vi "Comm visa sync.vi"(8 "error in (no error)":errorcluster, 10 "Command":u8[](array[numeric]), 11 "VISA in":refnum<visa-resource-name>="COM7") -> (0 "error out":errorcluster, 1 "sync info":string, 2 "Response":string, 3 "VISA out":refnum<visa-resource-name>)   [LabVIEW 2014, in "AISAS motor.lvclass"]
uses:
  AISAS motor.lvclass
  <vilib>/Instr/_visa.llb/VISA Flush IO Buffer Mask.ctl
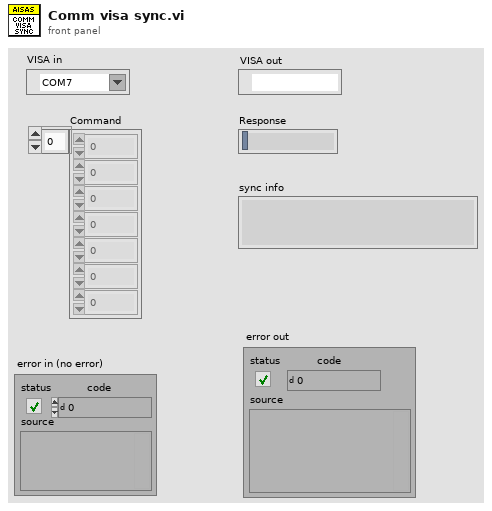
[diagram p1: front panel]
types:
  T1 = typedef "VISA Flush IO Buffer Mask.ctl" = u16
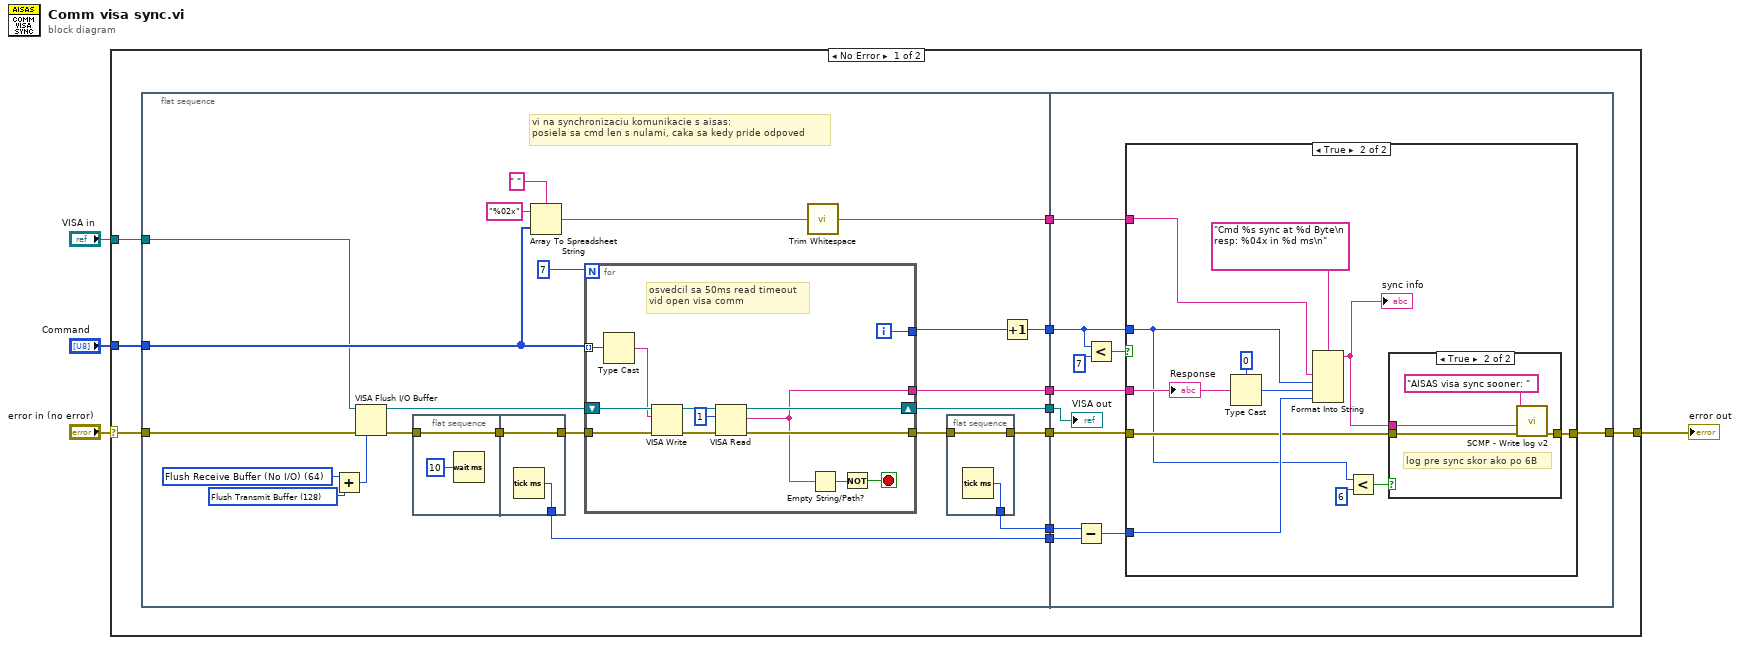
[diagram p0: block diagram]
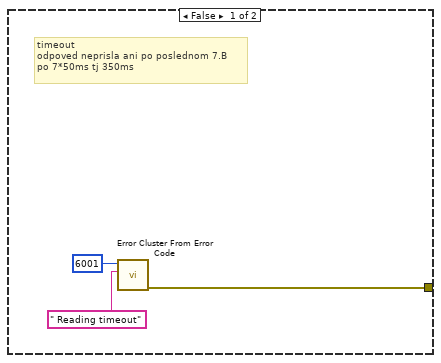
[diagram p2: hidden frame]
diagram:
  n1 = case shown="No Error" "error in (no error)" {
    selector: "error in (no error)" -> [w8 w89]
    tunnel: [w12 w89] -> w3
    tunnel: "Command" -> [w6 _]
    tunnel: "VISA in" -> [w5 _]
    frame No Error {
      n2 = flat-sequence {
        tunnel: [w38] -> w15
        tunnel: [w34] -> w14
        tunnel: [w36] -> w13
        tunnel: [w24] -> w11
        tunnel: [w33] -> w10
        tunnel: [w32] -> w9
        tunnel: w8 -> [w19]
        tunnel: [w27] -> w7
        tunnel: w6 -> [w26]
        tunnel: w5 -> [w16]
        tunnel: [w64] -> w12
        tunnel: w15 -> [w59]
        tunnel: w14 -> [w63]
        tunnel: w13 -> [w66]
        tunnel: w11 -> [w65]
        tunnel: w10 -> [w61]
        tunnel: w9 -> [w62]
        tunnel: w7 -> [w58]
        frame #0 {
          w21 = T1 128 items=["Flush Receive Buffer"=16, "Write Transmit Buffer to Device"=32, "Flush Receive Buffer (No I/O)"=64, "Flush Transmit Buffer"=128] ("y")
          w22 = T1 64 items=["Flush Receive Buffer"=16, "Write Transmit Buffer to Device"=32, "Flush Receive Buffer (No I/O)"=64, "Flush Transmit Buffer"=128] ("Mask")
          # "vi na synchronizaciu komunikacie s aisas:\nposiela sa cmd len s nulami, caka sa kedy pride odpoved"
          n3 = Add(x=w22, y=w21) -> (x+y=w20:T1)
          n4 = VISA Flush I/O Buffer(VISA resource name=w16, mask (16)=w20, error in (no error)=w19) -> (VISA resource name out=w17:refnum<visa-resource-name>, error out=w18:errorcluster)
          n5 = flat-sequence {
            tunnel: w18 -> [w42]
            tunnel: [w42] -> w23
            tunnel: [w44] -> w33
            tunnel: [w43] -> w31
            tunnel: w23 -> [w43]
            frame #0 {
              n6 = Wait (ms)(milliseconds to wait=u32 10) -> ()  [unwired: 1 out]
            }
            frame #1 {
              n7 = Tick Count (ms)() -> (millisecond timer value=w44:u32)
            }
          }
          n8 = Array To Spreadsheet String(delimiter (Tab)=" ", array=w26, 3:"%02x" ("format string")) -> (spreadsheet string=w28:string)
          n9 = for {
            N: 7 -> [_]
            shift-right: [w57] -> w38
            shift-left: w17 -> [w56]
            tunnel: [w49] -> w36
            tunnel: [w54] -> w25
            tunnel: [w55] -> w35
            tunnel: w31 -> [w47]
            tunnel: w26 -> [w45] mode=indexing
            i -> [w54]
            stop <- w48 stop-if-true
            # "osvedcil sa 50ms read timeout\nvid open visa comm"
            n10 = Type Cast(x=w45) -> (*(type *) &x=w46:string)  [unwired: 1 in]
            n11 = VISA Write(VISA resource name=w56, write buffer=w46, error in (no error)=w47) -> (VISA resource name out=w53:refnum<visa-resource-name>, error out=w52:errorcluster)  [unwired: 1 out]
            n12 = VISA Read(VISA resource name=w53, byte count=u32 1, error in (no error)=w52) -> (VISA resource name out=w57:refnum<visa-resource-name>, read buffer=w49:string, error out=w55:errorcluster)  [unwired: 1 out]
            n13 = Empty String/Path?(string/path=w49) -> (empty?=w50:bool)
            n14 = Not(x=w50) -> (.not. x?=w48:bool)
          }
          n15 = call <vilib>:"Trim Whitespace.vi"("string"=w28) -> ("trimmed string"=w27:string)  [unwired: 1 in]
          n16 = flat-sequence {
            tunnel: w35 -> [w40]
            tunnel: [w40] -> w34
            tunnel: [w39] -> w32
            frame #0 {
              n17 = Tick Count (ms)() -> (millisecond timer value=w39:u32)
            }
          }
          n18 = Increment(x=w25) -> (x+1=w24:i32)
        }
        frame #1 {
          n19 = Subtract(x=w62, y=w61) -> (x-y=w60:u32)
          n20 = Less?(x=w65, y=7) -> (x < y?=w67:bool)
          n21 = case shown="True" w67 {
            tunnel: w63 -> [_ w77]
            tunnel: [w69 w76] -> w64
            tunnel: w66 -> [_ w83]
            tunnel: w65 -> [_ w72]
            tunnel: w60 -> [_ w82]
            tunnel: w58 -> [_ w81]
            frame False {
              # "timeout\nodpoved neprisla ani po poslednom 7.B\npo 7*50ms tj 350ms"
              n22 = call <vilib>:"Error Cluster From Error Code.vi"("error message (\"\")"=" Reading timeout" ("error message (\"\")"), "error code (0)"=6001) -> ("error out"=w69:errorcluster)  [unwired: 7 in]
            }
            frame True {
              n23 = Type Cast(type=u32 0, x=w83) -> (*(type *) &x=w78:u32)
              n24 = Format Into String(format string="Cmd %s sync at %d Byte\n  resp: %04x in %d ms\n" ("read buffer"), w81, w72, w78, w82) -> (resulting string=w75:string)  [unwired: 2 in, 1 out]
              "sync info" <- w75
              n25 = Less?(x=w72, y=6) -> (x < y?=w73:bool)
              n26 = case shown="True" w73 {
                tunnel: w77 -> [w84 w88]
                tunnel: [w84 w87] -> w76
                tunnel: w75 -> [_ w86]
                frame False {
                  # "sync ok presne po 6B,\n neloguje sa nic"
                }
                frame True {
                  # "log pre sync skor ako po 6B"
                  n27 = call "SCMP - Write log v2.vi"("Error to log"=w88, "data to end"=w86, "data"="AISAS visa sync sooner: ") -> ("error out"=w87:errorcluster)  [unwired: 6 in, 2 out]
                }
              }
              "Response" <- w83
            }
          }
          "VISA out" <- w59
        }
      }
    }
    frame Error {
    }
  }
  "error out" <- w3
